vi "getChannelAtributes.vi"(5 "Ch Name 2":string[][](array[string]), 6 "amplitude":dbl[](array[numeric]), 7 "polarity":enum16{"Negative", "Positive"}[](array[ring]), 8 "Ch Name":string[](array[string]), 9 "Delay":T1[](array[typedef]) min=-999.0 max=999.0 format="%+.12f") -> (0 "Array 4":T1[](array[typedef]) min=-999.0 max=999.0 format="%+.12f", 1 "Array 2":T1[](array[typedef]) min=-999.0 max=999.0 format="%+.12f", 2 "Array":T1[](array[typedef]) min=-999.0 max=999.0 format="%+.12f", 3 "Array 3":dbl[](array[numeric]))   [LabVIEW 2013]
uses:
  DelayControl2.ctl
  <userlib>/_OpenG.lib/array/array.llb/Sort 2D Array (String)__ogtk.vi
panel:
  out "Sorted Pointers":i32[](array[numeric])
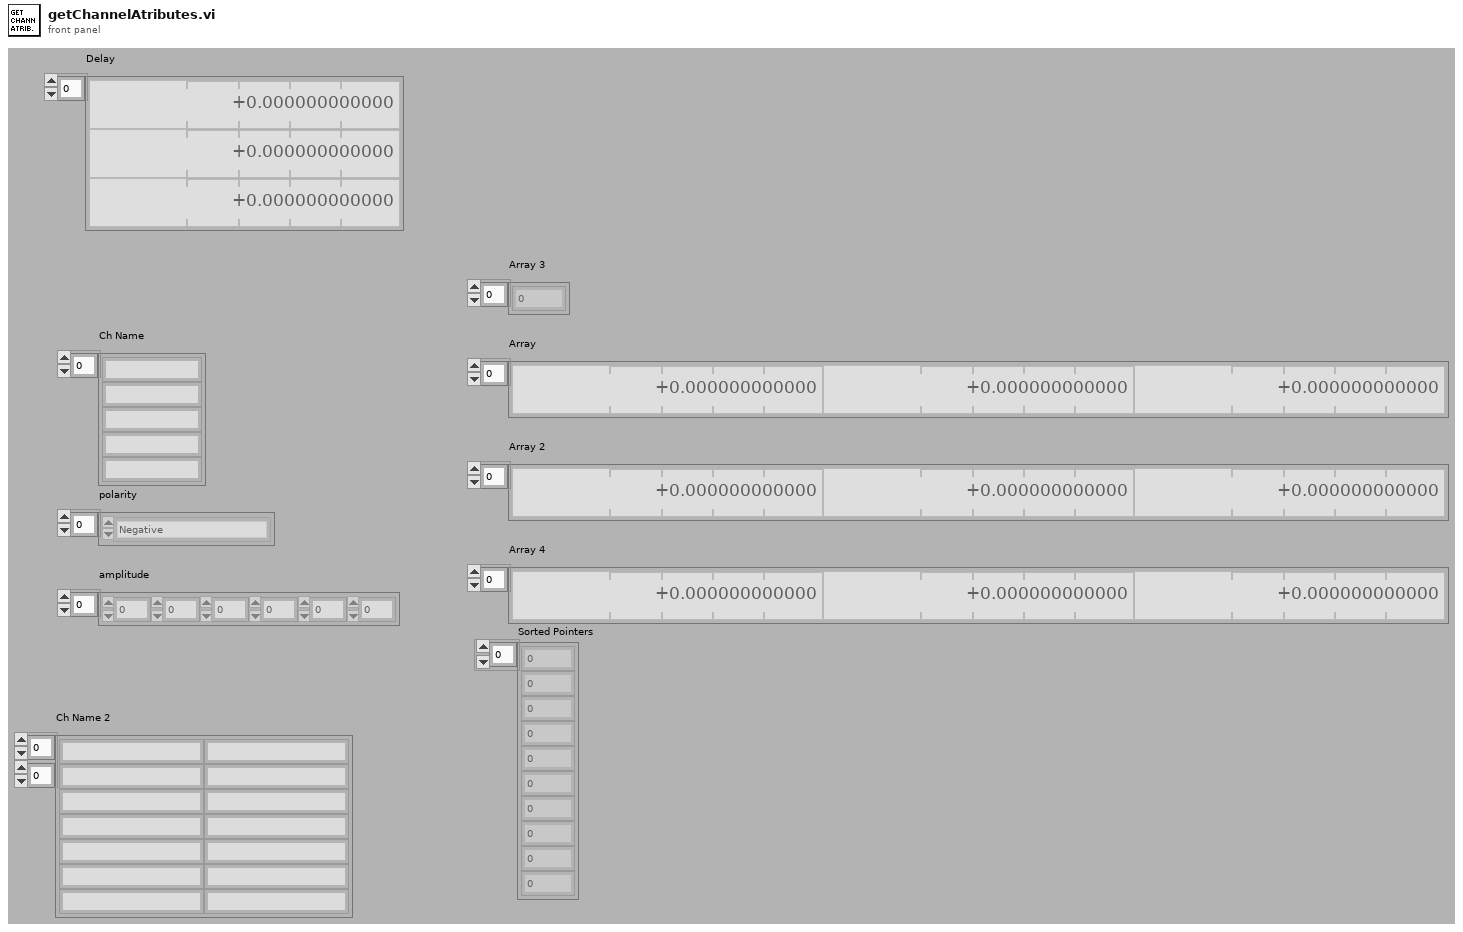
[diagram p1: front panel]
types:
  T1 = typedef "DelayControl2.ctl" = dbl
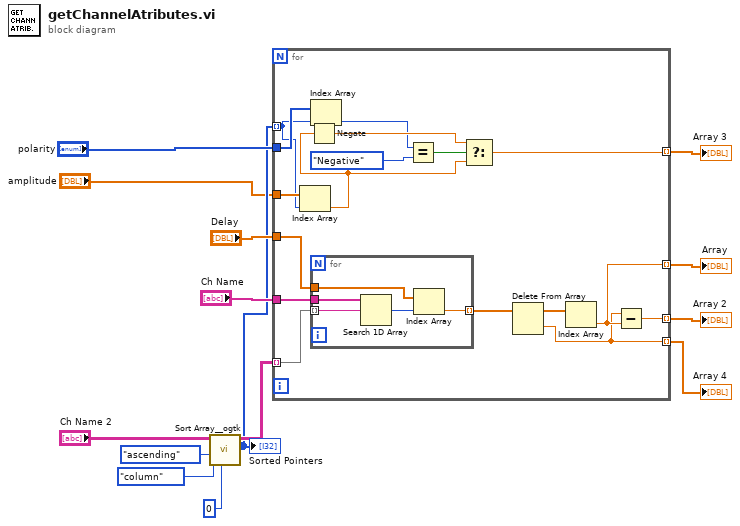
[diagram p0: block diagram]
diagram:
  n1 = call-poly <userlib>:"Sort Array__ogtk.vi"("Column/Row to Sort By"=u32 0, "Sort By in"=enum16{"row", "column"}."column", "Order"=enum16{"ascending", "descending"}."ascending", "Array in"="Ch Name 2") -> ("Sorted Pointers"=w2:i32[], "Sorted Array out"=w3:string[][])  [unwired: 4 in, 2 out]
  "Sorted Pointers" <- w2
  n2 = for {
    tunnel: w3 -> [w31] mode=indexing
    tunnel: "polarity" -> [w19]
    tunnel: "Ch Name" -> [w30]
    tunnel: "Delay" -> [w23]
    tunnel: [w24] -> w13 mode=indexing
    tunnel: [w21] -> w14 mode=indexing
    tunnel: [w25] -> w12 mode=indexing
    tunnel: [w20] -> w11 mode=indexing
    tunnel: w2 -> [w16] mode=indexing
    tunnel: "amplitude" -> [w17]
    n3 = Index Array(array=w17, index=w16) -> (element=w15:dbl)
    n4 = Negate(x=w15) -> (-x=w26:dbl)
    n5 = Index Array(array=w19, index=w16) -> (element=w18:enum16{"Negative", "Positive"})
    n6 = for {
      tunnel: w31 -> [w32] mode=indexing
      tunnel: w30 -> [w36]
      tunnel: w23 -> [w35]
      tunnel: [w33] -> w29 mode=indexing
      n7 = Search 1D Array(1D array=w36, element=w32) -> (index of element=w34:i32)  [unwired: 1 in]
      n8 = Index Array(array=w35, index=w34) -> (element=w33:T1)
    }
    n9 = Equal?(x=w18, y=enum16{"Negative", "Positive"}."Negative") -> (x = y?=w27:bool)
    n10 = Select(t=w26, s=w27, f=w15) -> (s? t:f=w25:dbl)
    n11 = Delete From Array(array=w29) -> (deleted portion=w20:T1, array with subset deleted=w22:T1[])  [unwired: 2 in]
    n12 = Index Array(array=w22) -> (element=w21:T1)  [unwired: 1 in]
    n13 = Subtract(x=w20, y=w21) -> (x-y=w24:T1)
  }
  "Array" <- w14
  "Array 2" <- w13
  "Array 3" <- w12
  "Array 4" <- w11
